vi "get connection settings.vi"(11 "connection server in":refnum<class "connection server.lvclass">) -> (2 "max allowed":i32, 3 "connection string":string)   [LabVIEW 2015, in "connection server.lvclass"]
uses:
  connection server.lvclass
  connection server.lvclass/connection server.ctl
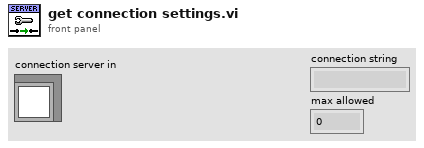
[diagram p1: front panel]
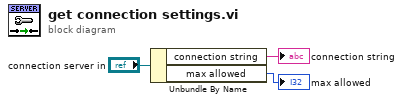
[diagram p0: block diagram]
diagram:
  n1 = Unbundle By Name("connection server in") -> ("connection string"=→"connection string":string, "max allowed"=→"max allowed":i32)
